vi "SaveGparhImage.vi"(4 "Option":T2={"JPG Quqlity(80)"=80, "PNG Comp(-1)"=-1}, 5 "Cut Border":T1={"Left"=1, "Up"=1, "Right"=1, "Down"=1}, 6 "Format":enum16{"JPG", "PNG", "BMP"}(ring), 7 "Image Path":path, 8 "error in (no error)":errorcluster caption="エラー入力（エラーなし）", 9 "BG Color":u32, 10 "Bit Depth":i32, 11 "WFGraph ref in":refnum<vi>) -> (0 "error out":errorcluster caption="エラー出力", 3 "WFGraph ref out":refnum<vi>)   [LabVIEW 2014]
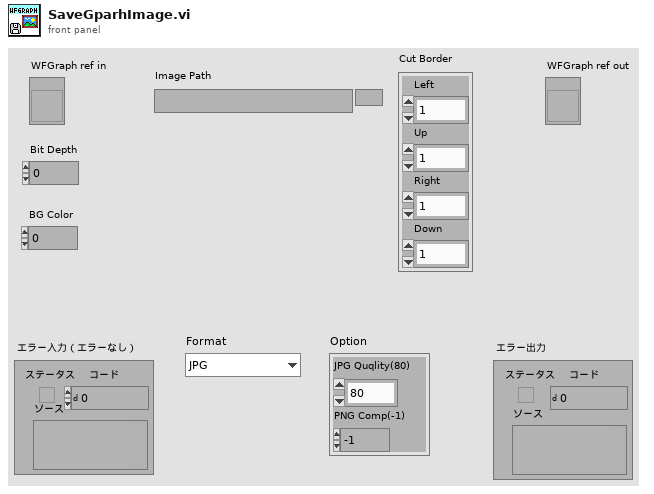
[diagram p1: front panel]
types:
  T1 = cluster{"Left":i16, "Up":i16, "Right":i16, "Down":i16}
  T2 = cluster{"JPG Quqlity(80)":i32, "PNG Comp(-1)":i32}
  T3 = typedef "imagedata.ctl" = cluster{"image type":i32, "image depth":i32, "image":u8[], "mask":u8[], "colors":u32[], "Rectangle":cluster{"left":i16, "top":i16, "right":i16, "bottom":i16}}
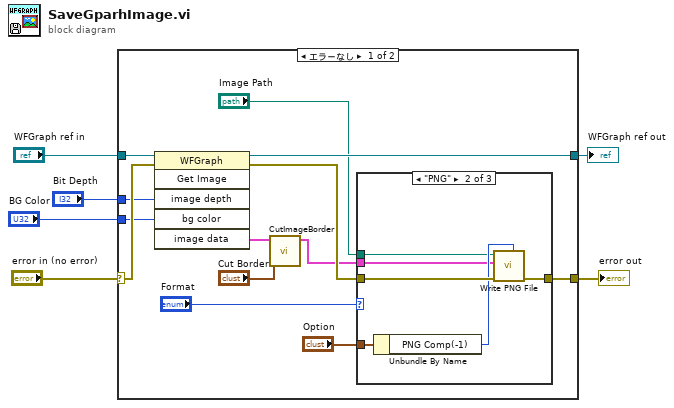
[diagram p0: block diagram]
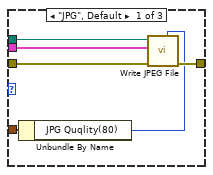
[diagram p2: hidden frame]
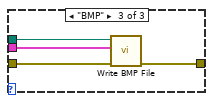
[diagram p3: hidden frame]
diagram:
  n1 = case shown="エラーなし" "error in (no error)" {
    selector: "error in (no error)" -> [w17 w37]
    tunnel: [w13 w37] -> w5
    tunnel: "WFGraph ref in" -> [w19 w36]
    tunnel: [w18 w36] -> w3
    tunnel: "Bit Depth" -> [w16 _]
    tunnel: "BG Color" -> [w15 _]
    frame No Error {
      n2 = invoke class="WFGraph" method="Get Image"(reference=w19, error in=w17, "image depth"=w16, "bg color"=w15) -> (reference out=w18:refnum<vi>, error out=w12:errorcluster, "image data"=w9:T3)  [unwired: 2 in, 3 out]
      n3 = call "CutImageBorder.vi"("削除枠幅"="Cut Border", "元画像"=w9) -> ("切抜き画像"=w8:T3)  [unwired: 9 in]
      n4 = case shown="\"PNG\"" "Format" {
        tunnel: [w25 w31 w32] -> w13
        tunnel: w12 -> [w24 w30 w35]
        tunnel: "Image Path" -> [w23 w27 w34]
        tunnel: w8 -> [w22 w26 w33]
        tunnel: "Option" -> [w21 w29 _]
        frame "JPG", Default {
          n5 = Unbundle By Name(w21) -> ("JPG Quqlity(80)"=w20:i32)
          n6 = call <vilib>:"Write JPEG File.vi"("quality (80)"=w20, "error in (no error)"=w24, "image data"=w22, "path to JPEG file"=w23) -> ("error out"=w25:errorcluster)  [unwired: 6 in, 1 out]
        }
        frame "PNG" {
          n7 = Unbundle By Name(w29) -> ("PNG Comp(-1)"=w28:i32)
          n8 = call <vilib>:"Write PNG File.vi"("compression (default)"=w28, "error in (no error)"=w30, "image data"=w26, "path to PNG file"=w27) -> ("error out"=w31:errorcluster)  [unwired: 6 in, 1 out]
        }
        frame "BMP" {
          n9 = call <vilib>:"Write BMP File.vi"("error in (no error)"=w35, "image data"=w33, "path to BMP file"=w34) -> ("error out"=w32:errorcluster)  [unwired: 7 in, 1 out]
        }
      }
    }
    frame Error {
    }
  }
  "error out" <- w5
  "WFGraph ref out" <- w3
